vi "load_config_svi.vi"(8 "Config Directory":path=path "D:/ParDates") -> (10 "Noff":u32 step=1, 12 "USED_FILTERS":u8[](array[numeric]), 14 "USED_LEDS":bool[][](array[boolean]), 15 "NPAT":u32, 16 "EXPT":dbl, 17 "BETWEEN_SCAN":u32, 18 "Non":u32=150 step=1, 19 "NSCAN":u32, 20 "Refnum VISA en sortie":refnum<visa-resource-name>="COM1", 21 "BIN":u16, 22 "Nstart":u32=30 step=1, 23 "ROMODE":u32, 24 "BETWEEN_PAT":u32, 25 "STAGE_SPEED":dbl, 26 "XYPOS":T1)   [LabVIEW 2013]
uses:
  <vilib>/Analysis/Matrix/Datatypes/RealMatrix.ctl
  <vilib>/Analysis/Matrix/NI_Matrix.lvlib
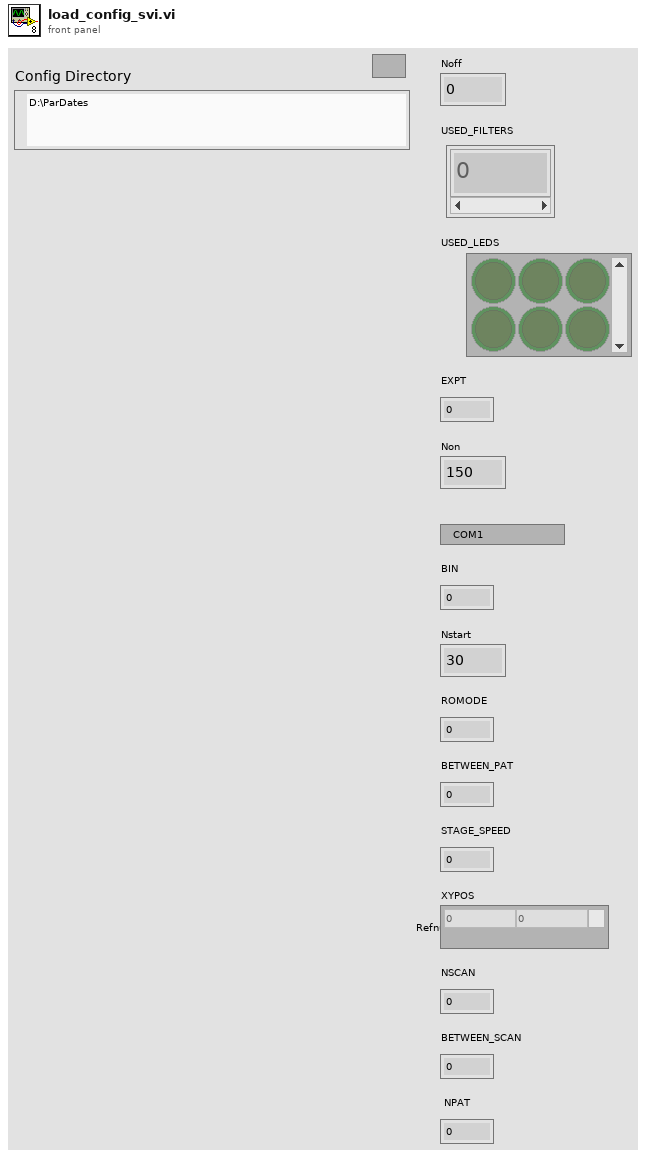
[diagram p1: front panel]
types:
  T1 = typedef "NI_Matrix.lvlib/RealMatrix.ctl" = dbl[][]
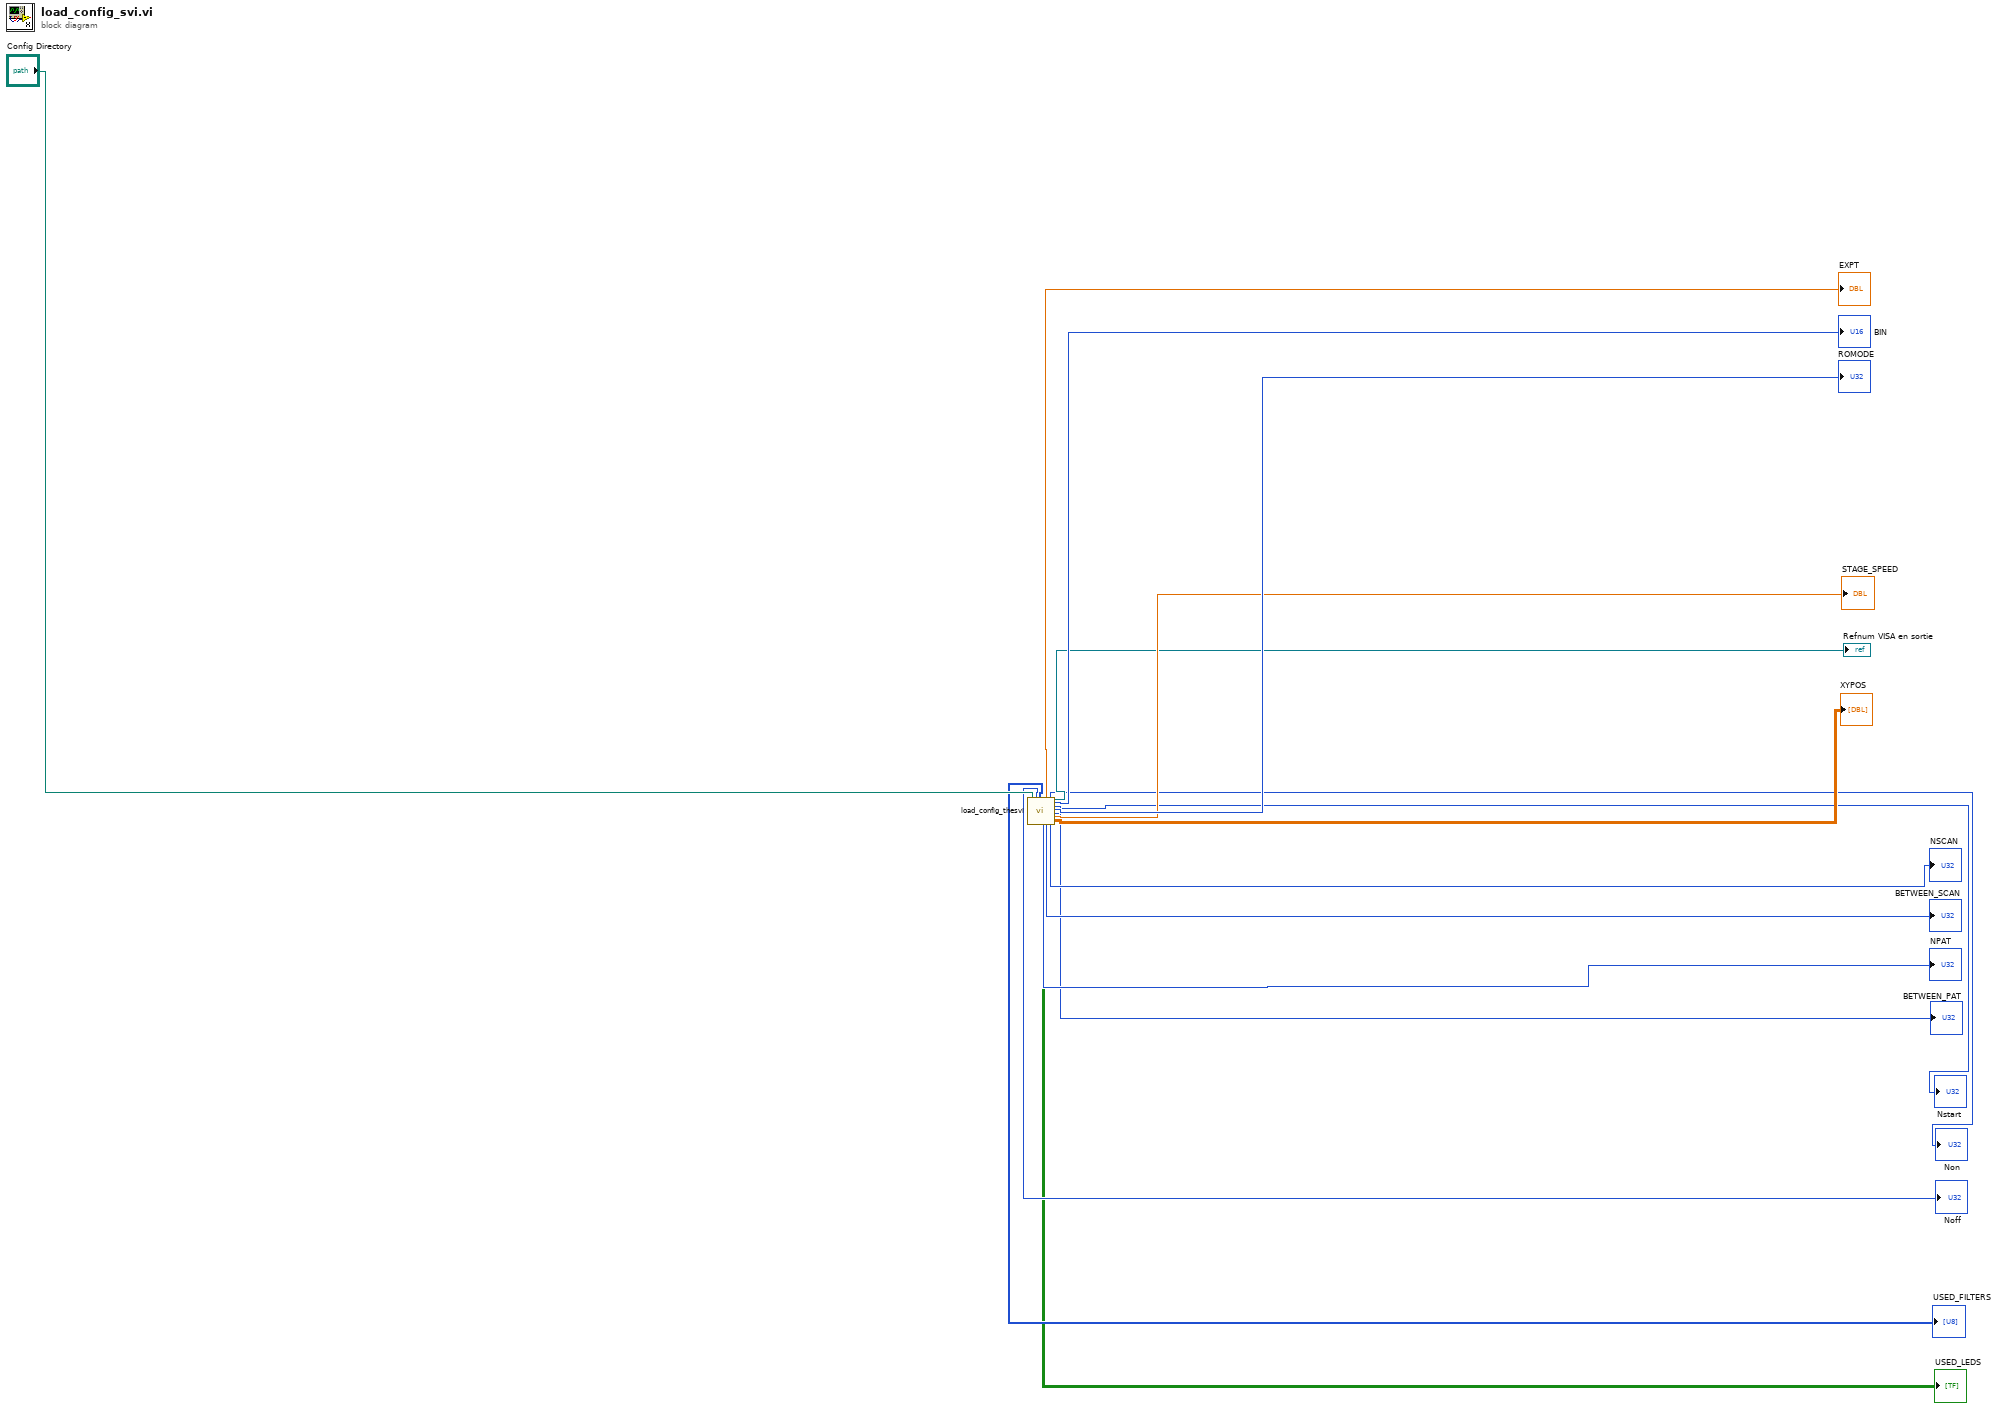
[diagram p0: block diagram]
diagram:
  n1 = call "load_config_thesvi.vi"("Config Directory"="Config Directory") -> ("Noff"=→"Noff":u32, "USED_FILTERS"=→"USED_FILTERS":u8[], "USED_LEDS"=→"USED_LEDS":bool[][], "NPAT"=→"NPAT":u32, "EXPT"=→"EXPT":dbl, "BETWEEN_SCAN"=→"BETWEEN_SCAN":u32, "Non"=→"Non":u32, "NSCAN"=→"NSCAN":u32, "Refnum VISA en sortie"=→"Refnum VISA en sortie":refnum<visa-resource-name>, "BIN"=→"BIN":u16, "Nstart"=→"Nstart":u32, "ROMODE"=→"ROMODE":u32, "BETWEEN_PAT"=→"BETWEEN_PAT":u32, "STAGE_SPEED"=→"STAGE_SPEED":dbl, "XYPOS"=→"XYPOS":T1)  [unwired: 12 in]
